vi "PathPlanner_TrajectoryState25_CopyWithTime.vi"(9 "TimeSeconds":dbl, 11 "PathPlannerState":T1={"TimeSeconds"=0.0, "LinearVelocity"=0.0, "Heading"={"VALUE"=0.0, "COS"=1.0, "SIN"=0.0}, "Constraints"={"MaxVelocityMps;"=0.0, "MaxAccelerationMpsSq;"=0.0, "MaxAngularVelRadPsEc;"=0.0, "MaxAngularAccRadPSecSq"=0.0, "Exists"=FALSE, "Unlimited"=FALSE, "NominalVoltageVolts"=12.0}, "DeltaPos"=0.0, "FieldSpeeds"={"vX"=0.0, "vY"=0.0, "vOmega"=0.0}, "pose"={"TRANSLATION"={"X"=0.0, "Y"=0.0}, "ROTATION"={"VALUE"=0.0, "COS"=1.0, "SIN"=0.0}}, "DeltaRot"={"VALUE"=0.0, "COS"=1.0, "SIN"=0.0}, "ModuleStates"=[], "WaypointRelPos"=0.0, "Feedforwards"={"accelerationsMPSSq"=[], "linearForcesNewtons"=[], "torqueCurrentsAmps"=[], "robotRelativeForcesXNewtons"=[], "robotRelativeForcesYNewtons"=[]}} {"ModuleStates"."SWERVE_DRIVE_MODULE_STATE"."Angle"."SIN" format="%13.4f"; "ModuleStates"."SWERVE_DRIVE_MODULE_STATE"."Angle"."COS" format="%13.4f"; "ModuleStates"."SWERVE_DRIVE_MODULE_STATE"."Angle"."VALUE" format="%13.4f"; "ModuleStates"."FieldAngle"."SIN" format="%13.4f"; "ModuleStates"."FieldAngle"."COS" format="%13.4f"; "ModuleStates"."FieldAngle"."VALUE" format="%13.4f"; "ModuleStates"."FieldPos"."Y" format="%14.3f"; "ModuleStates"."FieldPos"."X" format="%14.3f"; "DeltaRot"."SIN" format="%13.4f"; "DeltaRot"."COS" format="%13.4f"; "DeltaRot"."VALUE" format="%13.4f"; "pose"."ROTATION"."SIN" format="%13.4f"; "pose"."ROTATION"."COS" format="%13.4f"; "pose"."ROTATION"."VALUE" format="%13.4f"; "pose"."TRANSLATION"."Y" format="%14.3f"; "pose"."TRANSLATION"."X" format="%14.3f"; "FieldSpeeds"."vOmega" format="%10.3f"; "FieldSpeeds"."vY" format="%10.3f"; "FieldSpeeds"."vX" format="%10.3f"; "Heading"."SIN" format="%13.4f"; "Heading"."COS" format="%13.4f"; "Heading"."VALUE" format="%13.4f"}) -> (3 "StateWithNewTime":T1={"TimeSeconds"=0.0, "LinearVelocity"=0.0, "Heading"={"VALUE"=0.0, "COS"=1.0, "SIN"=0.0}, "Constraints"={"MaxVelocityMps;"=0.0, "MaxAccelerationMpsSq;"=0.0, "MaxAngularVelRadPsEc;"=0.0, "MaxAngularAccRadPSecSq"=0.0, "Exists"=FALSE, "Unlimited"=FALSE, "NominalVoltageVolts"=12.0}, "DeltaPos"=0.0, "FieldSpeeds"={"vX"=0.0, "vY"=0.0, "vOmega"=0.0}, "pose"={"TRANSLATION"={"X"=0.0, "Y"=0.0}, "ROTATION"={"VALUE"=0.0, "COS"=1.0, "SIN"=0.0}}, "DeltaRot"={"VALUE"=0.0, "COS"=1.0, "SIN"=0.0}, "ModuleStates"=[], "WaypointRelPos"=0.0, "Feedforwards"={"accelerationsMPSSq"=[], "linearForcesNewtons"=[], "torqueCurrentsAmps"=[], "robotRelativeForcesXNewtons"=[], "robotRelativeForcesYNewtons"=[]}} {"ModuleStates"."SWERVE_DRIVE_MODULE_STATE"."Angle"."SIN" format="%13.4f"; "ModuleStates"."SWERVE_DRIVE_MODULE_STATE"."Angle"."COS" format="%13.4f"; "ModuleStates"."SWERVE_DRIVE_MODULE_STATE"."Angle"."VALUE" format="%13.4f"; "ModuleStates"."FieldAngle"."SIN" format="%13.4f"; "ModuleStates"."FieldAngle"."COS" format="%13.4f"; "ModuleStates"."FieldAngle"."VALUE" format="%13.4f"; "ModuleStates"."FieldPos"."Y" format="%14.3f"; "ModuleStates"."FieldPos"."X" format="%14.3f"; "DeltaRot"."SIN" format="%13.4f"; "DeltaRot"."COS" format="%13.4f"; "DeltaRot"."VALUE" format="%13.4f"; "pose"."ROTATION"."SIN" format="%13.4f"; "pose"."ROTATION"."COS" format="%13.4f"; "pose"."ROTATION"."VALUE" format="%13.4f"; "pose"."TRANSLATION"."Y" format="%14.3f"; "pose"."TRANSLATION"."X" format="%14.3f"; "FieldSpeeds"."vOmega" format="%10.3f"; "FieldSpeeds"."vY" format="%10.3f"; "FieldSpeeds"."vX" format="%10.3f"; "Heading"."SIN" format="%13.4f"; "Heading"."COS" format="%13.4f"; "Heading"."VALUE" format="%13.4f"})   [LabVIEW 2019, in "PathPlanner24.lvlib"]
doc: "Get the state reversed, used for following a trajectory reversed with a differential drivetrain\n \nInputs: \n - trajectoryState - cluster - this trajectory state\n\nOutputs:\n - ReversedState- trajectorystate - The reversed state"
uses:
  PathPlanner24.lvlib
  TypeDef/PathPlannerTrajectoryState25.ctl
  <vilib>/Rock Robotics/WPI/ThirdParty/JAS_Junk/TrajLib/TypeDef/ROTATION2D.ctl
  TypeDef/PathPlannerPathConstraints.ctl
  <vilib>/Rock Robotics/WPI/ThirdParty/JAS_Junk/TrajLib/TypeDef/CHASSIS_SPEEDS.ctl
  <vilib>/Rock Robotics/WPI/ThirdParty/JAS_Junk/TrajLib/TypeDef/POSE2D.ctl
  <vilib>/Rock Robotics/WPI/ThirdParty/JAS_Junk/TrajLib/TypeDef/TRANSLATION2D.ctl
  TypeDef/PathPlannerSwerveModTrajState.ctl
  <vilib>/Rock Robotics/WPI/ThirdParty/JAS_Junk/TrajLib/TypeDef/SWERVE_DRIVE_MODULE_STATE.ctl
  TypeDef/PathPlannerDriveFeedFwds.ctl
  <vilib>/Rock Robotics/WPI/ThirdParty/JAS_Junk/TrajLib/Trajectory_Library.lvlib
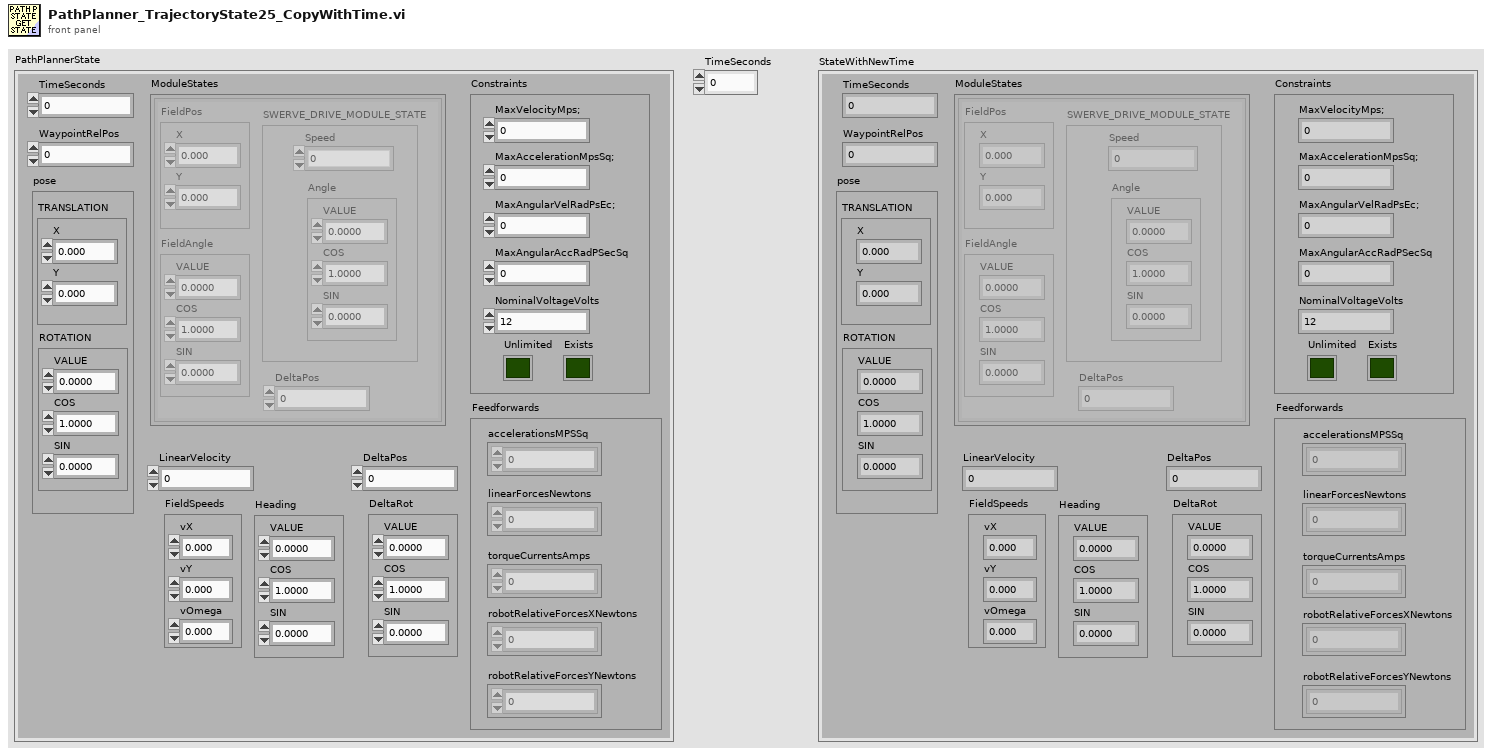
[diagram p1: front panel]
types:
  T1 = typedef "PathPlanner24.lvlib/PathPlannerTrajectoryState25.ctl" = cluster{"TimeSeconds":dbl, "LinearVelocity":dbl, "Heading":T2, "Constraints":T3, "DeltaPos":dbl, "FieldSpeeds":T4, "pose":T5, "DeltaRot":T2, "ModuleStates":T7[], "WaypointRelPos":dbl, "Feedforwards":T9}
  T2 = typedef "Trajectory_Library.lvlib/ROTATION2D.ctl" = cluster{"VALUE":dbl, "COS":dbl, "SIN":dbl}
  T3 = typedef "PathPlanner24.lvlib/PathPlannerPathConstraints.ctl" = cluster{"MaxVelocityMps;":dbl, "MaxAccelerationMpsSq;":dbl, "MaxAngularVelRadPsEc;":dbl, "MaxAngularAccRadPSecSq":dbl, "Exists":bool, "Unlimited":bool, "NominalVoltageVolts":dbl}
  T4 = typedef "Trajectory_Library.lvlib/CHASSIS_SPEEDS.ctl" = cluster{"vX":dbl, "vY":dbl, "vOmega":dbl}
  T5 = typedef "Trajectory_Library.lvlib/POSE2D.ctl" = cluster{"TRANSLATION":T6, "ROTATION":T2}
  T6 = typedef "Trajectory_Library.lvlib/TRANSLATION2D.ctl" = cluster{"X":dbl, "Y":dbl}
  T7 = typedef "PathPlanner24.lvlib/PathPlannerSwerveModTrajState.ctl" = cluster{"FieldPos":T6, "FieldAngle":T2, "DeltaPos":dbl, "SWERVE_DRIVE_MODULE_STATE":T8}
  T8 = typedef "Trajectory_Library.lvlib/SWERVE_DRIVE_MODULE_STATE.ctl" = cluster{"Speed":dbl, "Angle":T2}
  T9 = typedef "PathPlanner24.lvlib/PathPlannerDriveFeedFwds.ctl" = cluster{"accelerationsMPSSq":dbl[], "linearForcesNewtons":dbl[], "torqueCurrentsAmps":dbl[], "robotRelativeForcesXNewtons":dbl[], "robotRelativeForcesYNewtons":dbl[]}
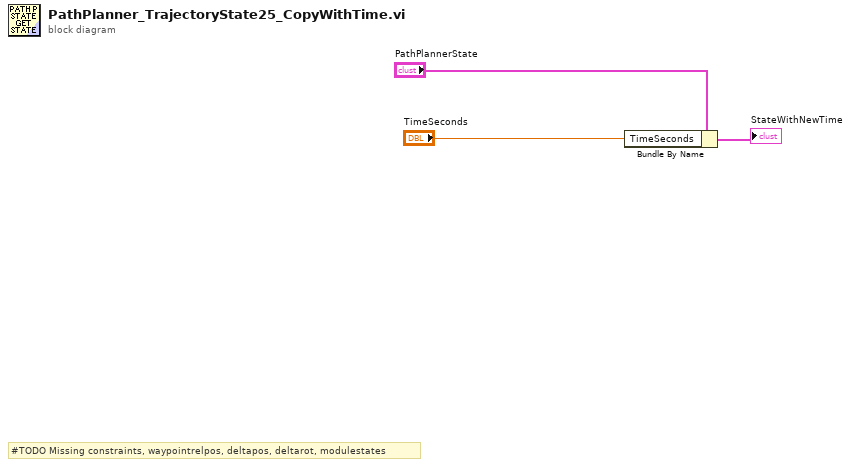
[diagram p0: block diagram]
diagram:
  # "#TODO Missing constraints, waypointrelpos, deltapos, deltarot, modulestates"
  n1 = Bundle By Name(cluster="PathPlannerState", "TimeSeconds"="TimeSeconds") -> (→"StateWithNewTime":T1)
